vi "CCIP.vi"(0 "Camera angle":dbl, 1 "zAvit":dbl, 3 "Processed Image":T2(plugin-control), 5 "Camera off set":dbl, 7 "Distance (from camera to target)":dbl, 9 "Compliting angle to 180":dbl, 12 "X center":dbl, 13 "Y center":dbl, 14 "Particle Scores":T1) -> (8 "Processed Image + aim markings":T2(plugin-control))   [LabVIEW 2012]
panel:
  in  "Convert Direction":u16(ring) items=["Nums to Pixels", "Pixel to Nums"]
  # "Shoot varubalse"
  # "Off set calculating"
  # "Drawing"
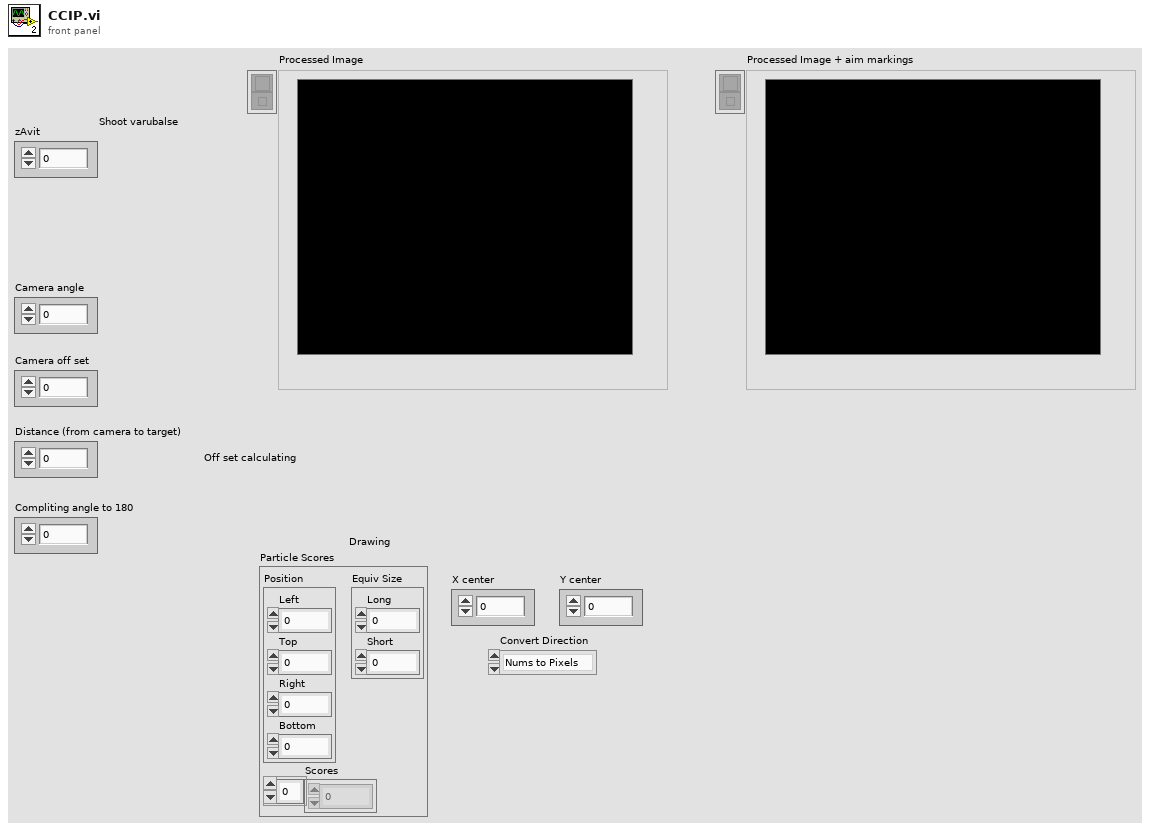
[diagram p1: front panel]
types:
  T1 = cluster{"Position":cluster{"Left":dbl, "Top":dbl, "Right":dbl, "Bottom":dbl}, "Scores":dbl[], "Equiv Size":cluster{"Long":dbl, "Short":dbl}}
  T2 = typedef "IMAQ Image.ctl" = refnum<image>
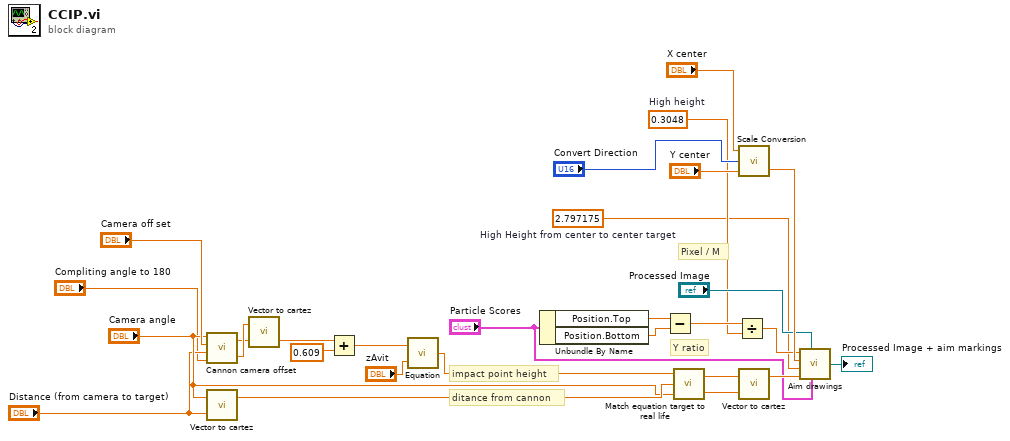
[diagram p0: block diagram]
diagram:
  w3 = 0.3048  # High height
  w2 = 2.797175  # High Height from center to center target
  # "Pixel / M"
  # "impact point height"
  # "ditance from cannon"
  # "Y ratio"
  n1 = call "Cannon camera offset.vi"("Compliting angle to 180"="Compliting angle to 180", "Distance (from camera)"="Distance (from camera to target)", "Offset (from center axis to camera lens)"="Camera off set", "Camera angle"="Camera angle") -> ("Angle (from cannon to target)"=w24:dbl, "Distance from cannon"=w23:dbl)
  n2 = call "Vector to cartez.vi"("Vector"="Distance (from camera to target)", "Angle [deg]"="Camera angle") -> ("Height"=w22:dbl)  [unwired: 1 out]
  n3 = call "Vector to cartez.vi"("Vector"=w23, "Angle [deg]"=w24) -> ("Length"=w1:dbl)  [unwired: 1 out]
  n4 = Add(x=w1, y=0.609) -> (x+y=w5:dbl)
  n5 = call "Equation.vi"("Distance"="zAvit", "zAvit"=w5) -> ("Calculated Height"=w7:dbl)
  n6 = Unbundle By Name("Particle Scores") -> ("Position.Top"=w10:dbl, "Position.Bottom"=w9:dbl)
  n7 = Subtract(x=w10, y=w9) -> (x-y=w8:dbl)
  n8 = call "Match equation target to real life.vi"("Camera angle"="Camera angle", "Height from camera"=w22, "Calculated height"=w7) -> ("Distance from Camera"=w18:dbl, "Angle on Camera"=w19:dbl)
  n9 = Divide(x=w8, y=w3) -> (x/y=w14:dbl)
  n10 = call "Scale Conversion.vi"("y in"="Y center", "Convert Direction"="Convert Direction", "x in"="X center") -> ("y out"=w16:dbl)  [unwired: 1 out]
  n11 = call "Vector to cartez.vi"("Vector"=w18, "Angle [deg]"=w19) -> ("Height"=w15:dbl)  [unwired: 1 out]
  n12 = call "Aim drawings.vi"("Particle Scores"="Particle Scores", "Processed Image"="Processed Image", "Calculated height [m]"=w15, "Center target position real life height [m]"=w2, "Center target position Y"=w16, "Y ratio"=w14) -> ("Processed Image + aim markings"=→"Processed Image + aim markings":T2)
